vi "GetLines.vi"(9 "delimiter":string="\n", 11 "String":string) -> (3 "Array":string[](array[string]))   [LabVIEW 2022 SP3]
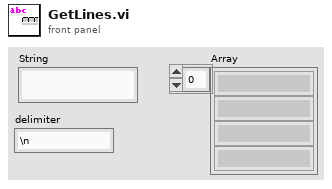
[diagram p1: front panel]
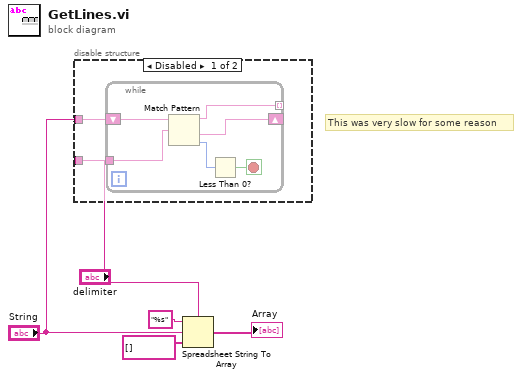
[diagram p0: block diagram]
diagram:
  # "This was very slow for some reason"
  n1 = disable-structure shown="Disabled" {
    disable-tunnel: "delimiter" -> [w7 _]
    disable-tunnel: "String" -> [w6 _]
    frame Disabled {
      n2 = while {
        shift-right: [w12] -> _
        shift-left: w6 -> [w13]
        tunnel: [w11] -> _ mode=indexing
        tunnel: w7 -> [w8]
        stop <- w9 stop-if-true
        n3 = Match Pattern(string=w13, regular expression=w8) -> (before substring=w11:string, after substring=w12:string, offset past match=w10:i32)  [unwired: 1 in, 1 out]
        n4 = Less Than 0?(x=w10) -> (x < 0?=w9:bool)
      }
    }
    frame Enabled {
    }
  }
  n5 = Spreadsheet String To Array(delimiter (Tab)="delimiter", format string="%s", spreadsheet string="String", array type (2D Dbl)=string[] []) -> (array=→"Array":string[])
